vi "setFPGAReference.vi"(10 "FPGAReference":refnum<k20>, 11 "ModbusPort1WriteFIFO in":refnum<class "ModbusPort1WriteFIFO.lvclass">) -> (3 "ModbusPort1WriteFIFO out":refnum<class "ModbusPort1WriteFIFO.lvclass">)   [LabVIEW 2016, in "ModbusPort1WriteFIFO.lvclass"]
uses:
  ModbusPort1WriteFIFO.lvclass
  ModbusPort1WriteFIFO.lvclass/ModbusPort1WriteFIFO.ctl
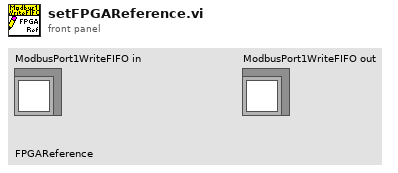
[diagram p1: front panel]
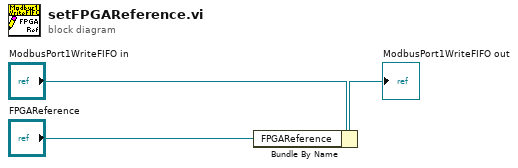
[diagram p0: block diagram]
diagram:
  n1 = Bundle By Name(cluster="ModbusPort1WriteFIFO in", "FPGAReference"="FPGAReference") -> (→"ModbusPort1WriteFIFO out":refnum<class "ModbusPort1WriteFIFO.lvclass">)
